vi "Comparison By Nth Element.vi"(9 "Element Index":u8, 10 "Person B":T1={"ID"=0, "Family Name"="Doe", "Given Name"="John", "Birth Date"=timestamp(3533142714.9178333 s since 1904-01-01)} {"Birth Date" format="%<%Y/%b/%d>T"}, 11 "Person A":T1={"ID"=0, "Family Name"="Smith", "Given Name"="John", "Birth Date"=timestamp(3533056306.0488334 s since 1904-01-01)} {"Birth Date" format="%<%Y/%b/%d>T"}) -> (3 "Swap?":bool)   [LabVIEW 2023]
doc: "This VI says that the two values should swap if Person A has a later birthday. If they have the same birthday, then they should swap if Person A has an alphabetically later name than Person B, checking last name first and then first name."
uses:
  Person Information.ctl
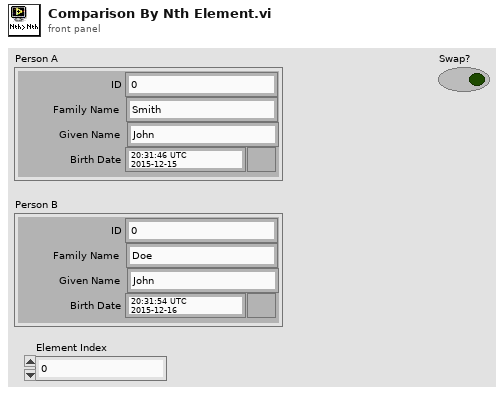
[diagram p1: front panel]
types:
  T1 = typedef "Person Information.ctl" = cluster{"ID":u32, "Family Name":string, "Given Name":string, "Birth Date":timestamp}
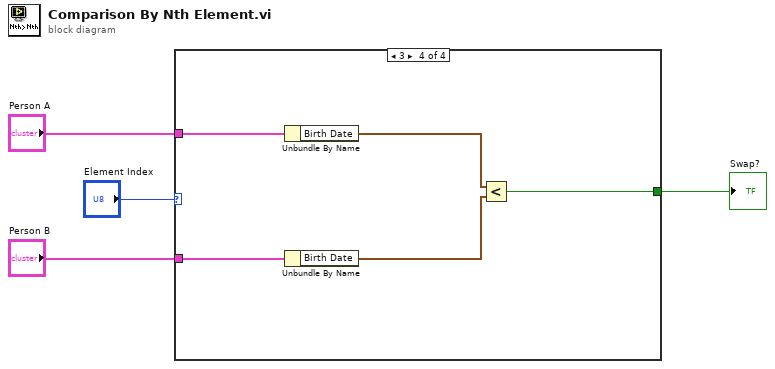
[diagram p0: block diagram]
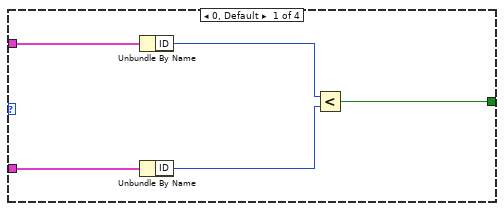
[diagram p2: hidden frame]
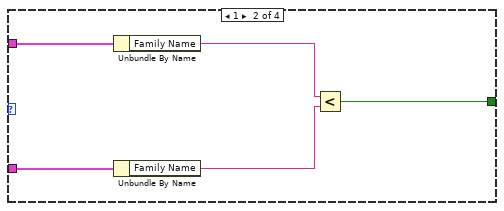
[diagram p3: hidden frame]
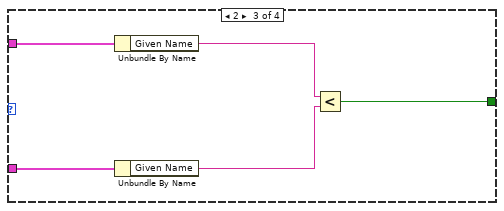
[diagram p4: hidden frame]
diagram:
  n1 = case shown="3" "Element Index" {
    tunnel: "Person B" -> [w9 w14 w19 w24]
    tunnel: "Person A" -> [w8 w13 w18 w23]
    tunnel: [w5 w10 w15 w20] -> w1
    frame 0, Default {
      n2 = Unbundle By Name(w8) -> ("ID"=w7:u32)
      n3 = Unbundle By Name(w9) -> ("ID"=w6:u32)
      n4 = Less?(x=w7, y=w6) -> (x < y?=w5:bool)
    }
    frame 1 {
      n5 = Unbundle By Name(w13) -> ("Family Name"=w12:string)
      n6 = Unbundle By Name(w14) -> ("Family Name"=w11:string)
      n7 = Less?(x=w12, y=w11) -> (x < y?=w10:bool)
    }
    frame 2 {
      n8 = Unbundle By Name(w18) -> ("Given Name"=w17:string)
      n9 = Unbundle By Name(w19) -> ("Given Name"=w16:string)
      n10 = Less?(x=w17, y=w16) -> (x < y?=w15:bool)
    }
    frame 3 {
      n11 = Unbundle By Name(w23) -> ("Birth Date"=w22:timestamp)
      n12 = Unbundle By Name(w24) -> ("Birth Date"=w21:timestamp)
      n13 = Less?(x=w22, y=w21) -> (x < y?=w20:bool)
    }
  }
  "Swap?" <- w1
